vi "get object descriptors.vi"(0 "i ref in":refnum<vi>, 2 "Object":string, 5 "error in (no error)":errorcluster) -> (14 "i ref out":refnum<vi>, 16 "selectors":string[](array[string]), 17 "Descriptors":string[](array[string]), 19 "error out":errorcluster)   [LabVIEW 2014, in "PTUtils.lvlib"]
uses:
  PTUtils.lvlib
  CS_Core/CSSystem/CoreDefs/CoreDefs.error_type.ctl
  CS_Core/CSSystem/CoreDefs/CoreDefs.error_severity.ctl
  CS_Core/CSSystem/CoreLib/CoreLib.byte array 2 string.vi
  CS_Core/CSSystem/CSSystemLib/CSSystemLib.lvlib
  CS_Core/CSSystem/CoreLib/CoreLib.lvlib
  CS_Core/BaseProcess/BaseProcess.lvlib
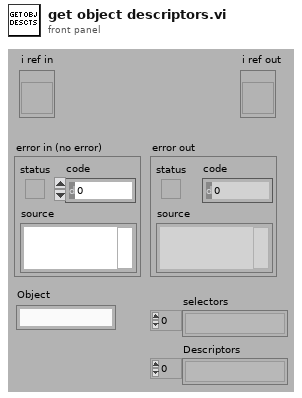
[diagram p1: front panel]
types:
  T1 = typedef "CoreDefs.error_severity.ctl" = enum16{"undefined", "information", "warning", "error", "fatal"}
  T2 = typedef "CoreDefs.error_type.ctl" = enum16{"no error", "can't load process", "can't unload process", "process does not exist", "can't install process", "can't remove process", "unknown function", "time out", "can't execute function", "duplicate queue name", "super not found", "caller queue invalid", "can't ping process", "unknown error", "VISA Error", "VISA timeout", "GPIB timeout", "GPIB error", "communication error", "data type mismatch", "can't read data from OPC server", "can't write data to OPC server", "OET error", "function not implemented", "process already exists", "invalid Shared Variable name", "error writing Shared Variable", "error reading Shared Variable", "invalid client name", "corrupt database", "unknown class", "call not authorized", "parameter out of range", "OET timeout: can't get data to modify", "invalid queue name", "requested operation incompatible with current state", "event undefined", "event disabled", "state undefined", "caller is not a friend", "EventBuilder: bad eventID", "EventBuilder: no DAQ devices", "a thread must not stop itself", "UNUSED ELEMENT4", "DiscArchiver: eventData incomplete", "DiscArchiver: eventData does not belong to run", "DiscArchiver: can't open file", "DiscArchiver: can't write to file", "DiscArchiver: available disc space low", "can't acquire semaphore", "error reading data from database", "notifier object is not existing", "can't register process", "can't unregister process", "illegal event type", "object disabled", "object already exists", "can't change state", "Instrument not found", "no connection to remote node", "invalid reference", "N/A", "UNUSED ELEMENT 1", "element not found", "illegal TCP/IP connection detected", "object does not exist", "invalid access ID", "unknown CS system", "invalid privilige", "unsupported data type", "unsupported server type", "IO server already exists", "Shared Variable already exists"}
  T3 = enum16{"simple", "synchronous", "asynchronous", "notification"}
  T4 = typedef "CoreDefs.call_type.ctl" = cluster{"Object":string, "Selector":string, "CallType":enum16{"simple", "synchronous", "asynchronous"}, "Async Object":string, "Async Selector":string, "Data Descriptor":T5, "Data":T6, "Error #":i32, "Expire":u32}
  T5 = typedef "BaseProcess.lvlib/BaseProcess.descriptor string definition.ctl" = string
  T6 = typedef "CoreDefs.rawDataType.ctl" = i8[]
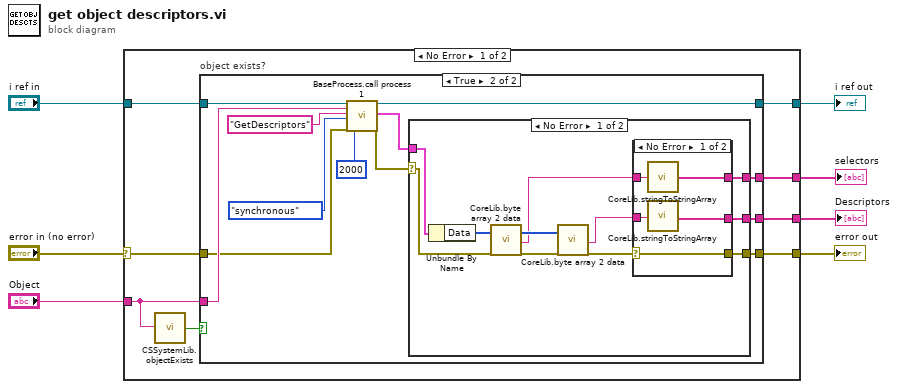
[diagram p0: block diagram]
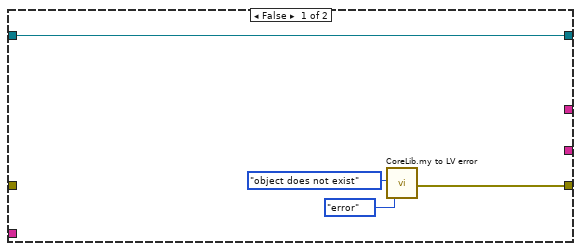
[diagram p2: hidden frame]
diagram:
  n1 = case shown="No Error" "error in (no error)" {
    selector: "error in (no error)" -> [w13 w50]
    tunnel: "i ref in" -> [w15 w51]
    tunnel: "Object" -> [w10 _]
    tunnel: [w14 w51] -> w5
    tunnel: [w12 w50] -> w4
    tunnel: [w9 _] -> w2
    tunnel: [w8 _] -> w1
    frame No Error {
      n2 = call "CSSystemLib.objectExists.vi"("name"=w10) -> ("obj exists"=w11:bool)
      n3 = case "object exists?" shown="True" w11 {
        tunnel: w15 -> [w19 w29]
        tunnel: w10 -> [_ w28]
        tunnel: [w19 w20] -> w14
        tunnel: w13 -> [_ w27]
        tunnel: [w18 w24] -> w12
        tunnel: [_ w22] -> w9
        tunnel: [_ w21] -> w8
        frame False {
          n4 = call "CoreLib.my to LV error.vi"("ErrorTypes"=CoreDefs.error_type."object does not exist", "severityLevel"=CoreDefs.error_severity."error") -> ("myErrorCluster"=w18:errorcluster)  [unwired: 16 in, 1 out]
        }
        frame True {
          n5 = call "BaseProcess.call process 1.vi"("i ref in"=w29, "Object"=w28, "Selector"="GetDescriptors", "CallType"=T3."synchronous", "error in (no error)"=w27, "timeout (ms)"=2000) -> ("i ref out"=w20:refnum<vi>, "call cluster out"=w26:T4, "error out"=w25:errorcluster)  [unwired: 11 in]
          n6 = case shown="No Error" w25 {
            selector: w25 -> [w38 w49]
            tunnel: w26 -> [w42 _]
            tunnel: [w32 w49] -> w24
            tunnel: [w34 _] -> w22
            tunnel: [w33 _] -> w21
            frame No Error {
              n7 = Unbundle By Name(w42) -> ("Data"=w41:T6)
              n8 = call-poly "CoreLib.byte array 2 data.vi"("byteArray"=w41, "error in (no error)"=w38) -> ("byteArray out"=w40:T6, "string"=w36:string, "error out"=w39:errorcluster)  [unwired: 15 in]
              n9 = call-poly "CoreLib.byte array 2 data.vi"("byteArray"=w40, "error in (no error)"=w39) -> ("string"=w35:string, "error out"=w37:errorcluster)  [unwired: 15 in, 1 out]
              n10 = case shown="No Error" w37 {
                selector: w37 -> [w47 w48]
                tunnel: [w47 w48] -> w32
                tunnel: w36 -> [w46 _]
                tunnel: w35 -> [w45 _]
                tunnel: [w43 _] -> w34
                tunnel: [w44 _] -> w33
                frame No Error {
                  n11 = call "CoreLib.stringToStringArray.vi"("String"=w46) -> ("Array"=w43:string[])
                  n12 = call "CoreLib.stringToStringArray.vi"("String"=w45) -> ("Array"=w44:string[])
                }
                frame Error {
                }
              }
            }
            frame Error {
            }
          }
        }
      }
    }
    frame Error {
    }
  }
  "error out" <- w4
  "i ref out" <- w5
  "selectors" <- w2
  "Descriptors" <- w1
